vi "Init.vi"(8 "error in (no error)":errorcluster, 11 "uService Template in":refnum<class "Error Manager.lvclass">) -> (0 "error out":errorcluster, 3 "uService Template out":refnum<class "Error Manager.lvclass">)   [LabVIEW 2026, in "TALOS.lvlib" / "Error Manager.lvlib" / "Error Manager.lvclass"]
uses:
  Error Manager.lvclass
  C:/LabVIEW Code/TALOS/talos/Ancestor/Ancestor/Ancestor.lvclass
  C:/LabVIEW Code/TALOS/talos/Father of all uServices/Father of all uServices/Father of all uServices.lvclass
  Error Manager.lvclass/Error Manager.ctl
  Ancestor/Ancestor/Ancestor.lvclass/Ancestor.ctl
  Father of all uServices/Father of all uServices/Father of all uServices.lvclass/Father of all uServices.ctl
  Ancestor/Ancestor/Infinite Message Selector.ctl
  Error Manager Consumer Case Selector.ctl
  Read Distributed flag.vi
  Ancestor/Ancestor/Read ID.vi
  Support VIs/Generate Error.vi
  FGV/Error Memory/Get Error Description.vi
  Support VIs/Get PC name.vi
  Support VIs/Get Class Name.vi
  <vilib>/Utility/error.llb/Clear Errors.vi
  FGV/Error Memory/Error Memory Core.vi
  <vilib>/AdvancedString/Delimited String to 1D String Array.vi
  <vilib>/AdvancedString/Delimited String to 1D String Array (string).vi
  Support VIs/Circus Root Path.vi
  FGV/Error Memory/Error Crt Lvl checker.vi
  FGV/Error Memory/Error Memory Core.vi/40c8088d-b597-4017-91af-faa98e00292e.vi
  FGV/Error Memory/Error Memory Core.vi/d4a3ab98-063c-4e44-b43d-fbdcfe6c2be2.vi
  Support VIs/Global Memory.vi
  <vilib>/Utility/LVClass/Get LV Class Name.vi
  Support VIs/Is in Packed Library.vi
  Support VIs/TALOS Root path.vi
  Support VIs/Read CSV worksheet.vi
  Support VIs/Global Constants.vi
  <vilib>/Utility/error.llb/General Error Handler.vi
  Support VIs/Error Log.vi
  Ancestor/Ancestor/Ancestor.lvclass
  <vilib>/Comparison/Equal/Equal Functor/Equal Functor.lvclass
  TALOS.lvlib
  Father of all uServices/Father of all uServices/Father of all uServices.lvclass
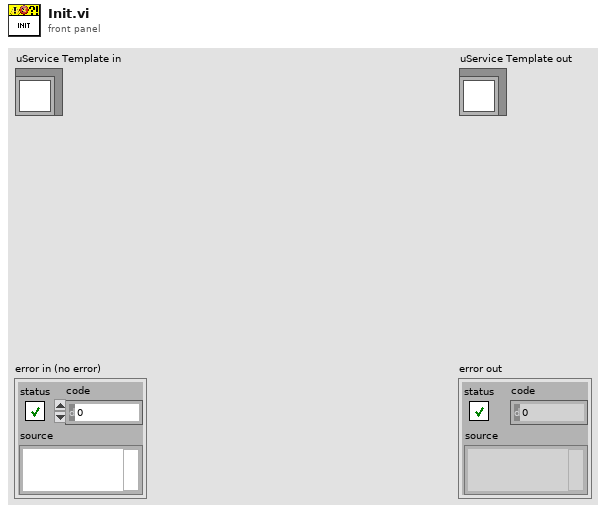
[diagram p1: front panel]
types:
  T1 = typedef "TALOS.lvlib/Error Manager.lvlib/Error Manager.lvclass/Error Manager Consumer Case Selector.ctl" = enum16{"Digest Error", "Dismiss Error", "Dismiss All", "Show Error Details", "Filter out Errors", "Clear Filters", "Check Distributed Mngr Status"}
  T2 = typedef "TALOS.lvlib/Ancestor.lvlib/Ancestor.lvclass/Infinite Message Selector.ctl" = enum16{"Start", "Stop", "Check", "Flush (Stop all)", "Init"}
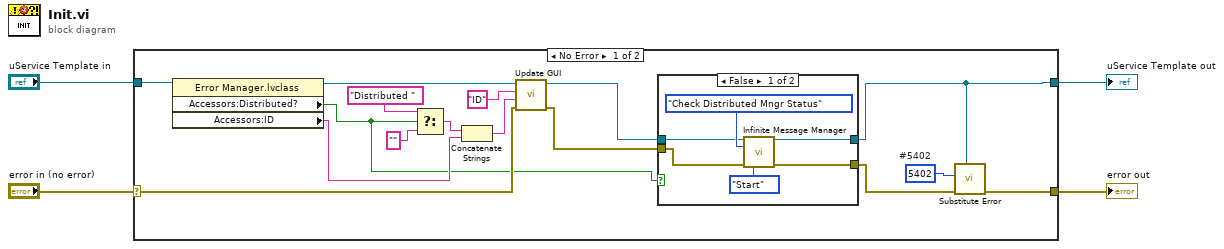
[diagram p0: block diagram]
diagram:
  n1 = case shown="No Error" "error in (no error)" {
    selector: "error in (no error)" -> [w11 w29]
    tunnel: "uService Template in" -> [w12 w30]
    tunnel: [w6 w30] -> w4
    tunnel: [w10 w29] -> w3
    frame No Error {
      w20 = 5402  # #5402
      n2 = property class="Error Manager.lvclass"(reference=w12) -> (reference out=w19:refnum<class "Error Manager.lvclass">, "Accessors:Distributed?"=w7:bool, "Accessors:ID"=w14:string)  [unwired: 1 in, 1 out]
      n3 = Select(t="Distributed ", s=w7, f="") -> (s? t:f=w15:string)
      n4 = Concatenate Strings(w15, w14) -> (w13:string)
      n5 = call "Update GUI.vi"("error in (no error)"=w11, "Data"=w13, "GUI Item Name"="ID", "uService Template in"=w19) -> ("error out"=w8:errorcluster, "uService Template out"=w9:refnum<class "Error Manager.lvclass">)  [unwired: 6 in]
      n6 = case shown="False" w7 {
        tunnel: [w24 w28] -> w5
        tunnel: [w23 w27] -> w6
        tunnel: w9 -> [w22 w27]
        tunnel: w8 -> [w21 w28]
        frame False {
          n7 = call-dynamic "Infinite Message Manager.vi"("Father of all uServices in"=w22, "Consumer Case Selector"=Error_Manager_Consumer_Case_Selector."Check Distributed Mngr Status" ("ErrMgr Case Selector"), "error in (no error)"=w21, "Infinite Message Selector"=Infinite_Message_Selector."Start") -> ("Father of all uServices out"=w23:refnum<class "Error Manager.lvclass">, "error out"=w24:errorcluster)  [unwired: 9 in, 1 out]
        }
        frame True {
        }
      }
      n8 = call "Substitute Error.vi"("LabVIEW Object"=w6, "error in (no error)"=w5, "Error Code"=w20) -> ("error out"=w10:errorcluster)  [unwired: 8 in]
    }
    frame Error {
    }
  }
  "error out" <- w3
  "uService Template out" <- w4
